vi "Kinesis - MPZ601 - Connect.vi"() -> ()   [LabVIEW 2012]
uses:
  U:/Kinesis LabVIEW Website Examples/Thorlabs.MotionControl.Controls.dll
  Thorlabs.MotionControl.Controls.dll
panel:
  in  "ChannelNumber":sgl=1.0
  in  "SerialNumber":string
  in  "?":bool
  in  "ModularPiezoControl":refnum<k24>(container)
  # "Notes:"
  # "- Ensure that the appropriate .DLLs are copied into your Project Folder. Check that the correct bit type are used depending on your version of LabVIEW\ni.e. 32-bit or 64-bit.\n\n\n\n\n\n\n\n\n\n\n\n\n\n\n- Open the example VI through the LabVIEW Project Explorer to correctly load the User Interface from Thorlabs.MotionControl.Controls.dll."
  # "Thorlabs Hardware: MPZ601 Rack Module 2-Ch Piezoelectric Controller With Feedback\nhttps://www.thorlabs.com/newgrouppage9.cfm?objectgroup_id=1185&pn=MPZ601#1185\n\nDescription: This VI will enable you to connect to & safely disconnect from the MPZ601 controller.\n\nInstructions: \n1) Connect your MPZ601 to your MMR601 Rack Module in any available bay.\n2) Connect the system to your control PC & power the device. For full device setup, the device product manual can be found on our website here. - https://www.thorlabs.com/thorproduct.cfm?partnumber=MPZ601\n3) Enter the device serial number below.\n4) Select the appropriate Channel \n4) Click 'Run' in the LabVIEW Toolbar.\n6) To end the VI, click 'END' to safely disconnect the device."
  # "Example Image of .NET Controller - VI opened via Project Explorer/ not opened via Project Explorer"
  # "VI Not Opened via Project Explorer"
  # "VI Opened via Project Explorer"
  # "- To explore the range of methods available, please visit the .NET API, included with your Kinesis software.\n\n- For tips on building your own VIs with Thorlabs Motion Control Hardware, please see our LabVIEW Guide here.\nhttps://www.thorlabs.com/newgrouppage9.cfm?objectgroup_id=10285"
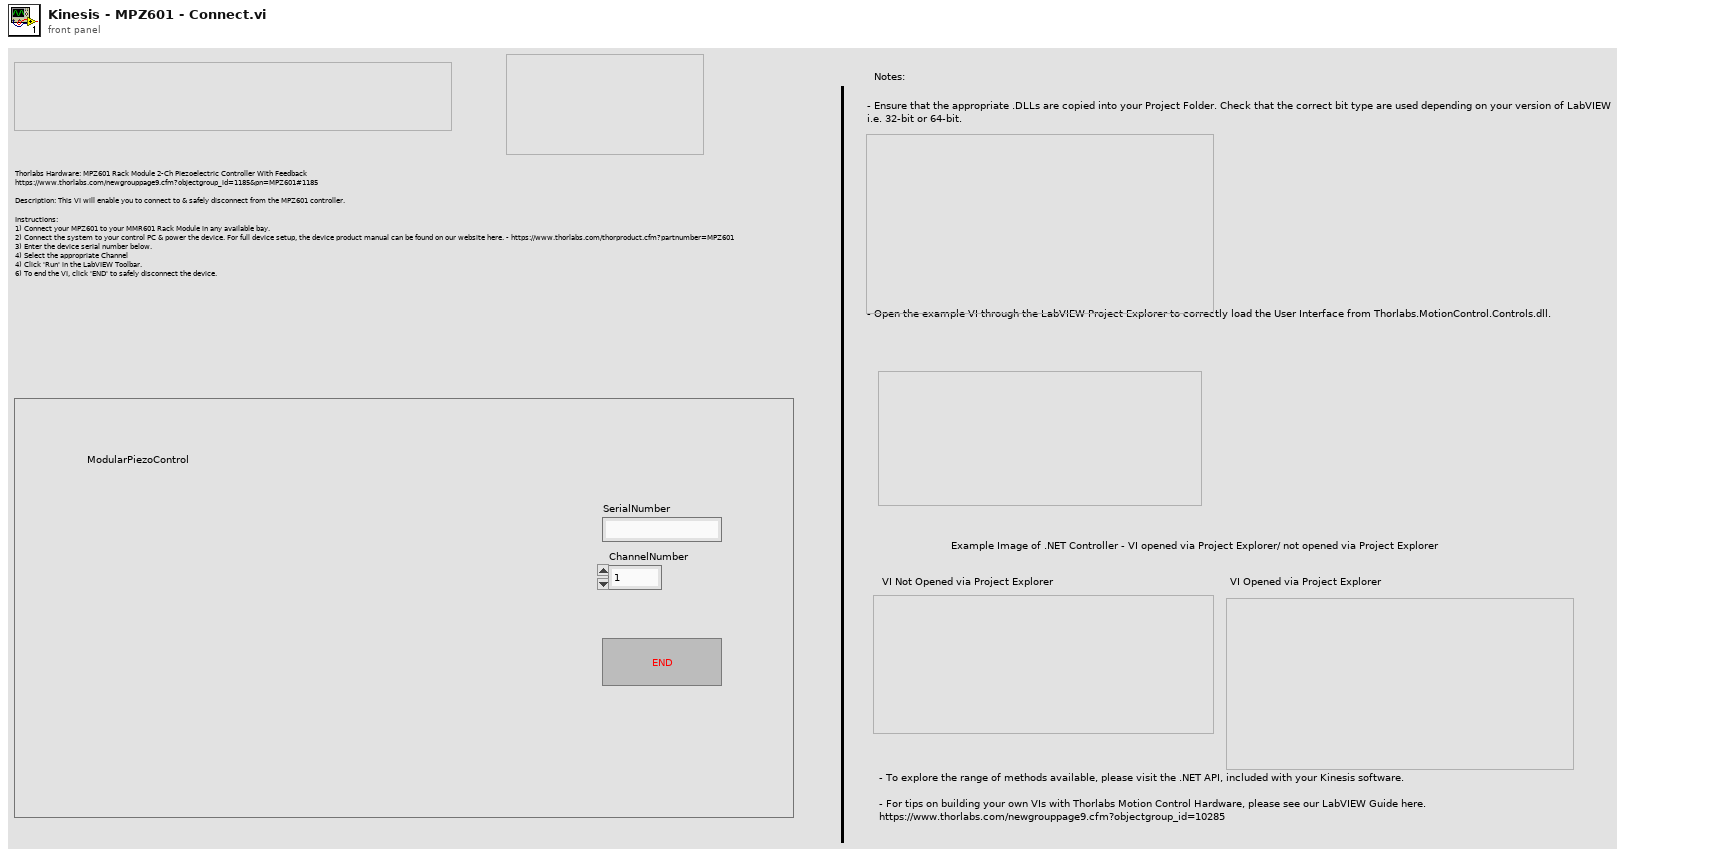
[diagram p1: front panel]
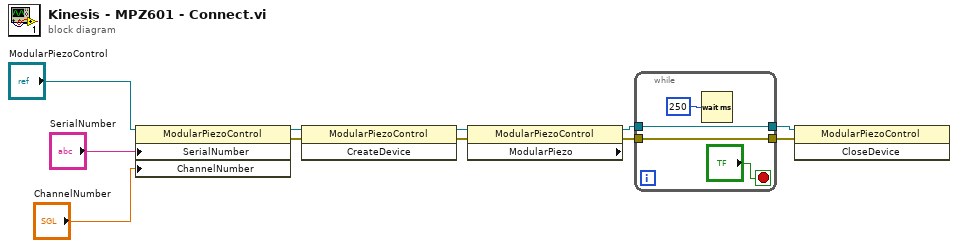
[diagram p0: block diagram]
diagram:
  n1 = property class="ModularPiezoControl"(reference="ModularPiezoControl", "SerialNumber"="SerialNumber", "ChannelNumber"="ChannelNumber") -> (reference out=w9:refnum<k24>, error out=w4:errorcluster)  [unwired: 1 in]
  n2 = invoke class="ModularPiezoControl" method="CreateDevice"(reference=w9, error in=w4) -> (reference out=w11:refnum<k24>, error out=w3:errorcluster)  [unwired: 1 in, 1 out]
  n3 = property class="ModularPiezoControl" props=["ModularPiezo"](reference=w11, error in=w3) -> (reference out=w5:refnum<k24>, error out=w2:errorcluster)  [unwired: 1 out]
  n4 = while {
    tunnel: [w14] -> w6
    tunnel: w5 -> [w14]
    tunnel: w2 -> [w12]
    tunnel: [w12] -> w1
    stop <- "?" stop-if-true
    n5 = Wait (ms)(milliseconds to wait=u32 250) -> ()  [unwired: 1 out]
  }
  n6 = invoke class="ModularPiezoControl" method="CloseDevice"(reference=w6, error in=w1) -> ()  [unwired: 1 in, 3 out]
